vi "Initialize Master.vi"(8 "error in":errorcluster, 11 "TCP master in":refnum<class "TCP Master.lvclass">) -> (0 "error out":errorcluster, 3 "TCP master out":refnum<class "TCP Master.lvclass">)   [LabVIEW 2013, in "Modbus Library - Advance.lvlib" / "TCP Master.lvclass"]
doc: "Opens a TCP connection to the address and port stored in the class."
uses:
  TCP Master.lvclass
  TCP Master.lvclass/TCP Master.ctl
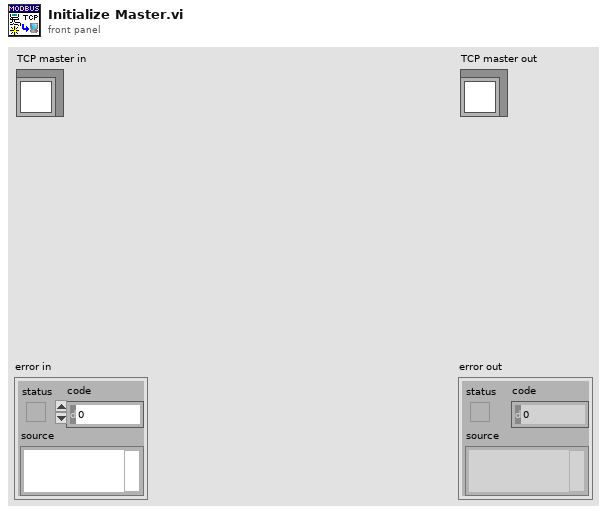
[diagram p1: front panel]
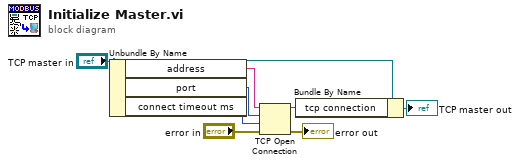
[diagram p0: block diagram]
diagram:
  n1 = Unbundle By Name("TCP master in") -> ("address"=w8:string, "port"=w7:u16, "connect timeout ms"=w1:i32)
  n2 = TCP Open Connection(address=w8, remote port or service name=w7, timeout ms (60000)=w1, error in (no error)="error in") -> (connection ID=w3:refnum<k5>, error out=→"error out":errorcluster)  [unwired: 1 in]
  n3 = Bundle By Name(cluster="TCP master in", "tcp connection"=w3) -> (→"TCP master out":refnum<class "TCP Master.lvclass">)
